vi "Write Background Mode.vi"(5 "Background Mode":enum16{"Stretch", "Center", "Tile"}(ring), 9 "Pane in":refnum<class "Pane.lvclass">) -> (3 "Pane out":refnum<class "Pane.lvclass">)   [LabVIEW 2014, in "Pane.lvclass"]
uses:
  Pane.lvclass
  Pane.lvclass/Pane.ctl
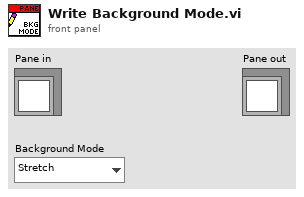
[diagram p1: front panel]
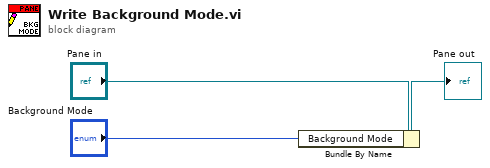
[diagram p0: block diagram]
diagram:
  n1 = Bundle By Name(cluster="Pane in", "Background Mode"="Background Mode") -> (→"Pane out":refnum<class "Pane.lvclass">)
